vi "Set AI Channel Scale Offset (Public).vi"(7 "AI":T1=enum."DrvrVoltage_AI", 8 "error in (no error)":errorcluster, 9 "ScaleOffset":dbl, 10 "IOName":string, 11 "DAQ":refnum<class "DAQ.lvclass">) -> (0 "error out":errorcluster, 3 "DAQ":refnum<class "DAQ.lvclass">)   [LabVIEW 2017, in "DAQ.lvclass"]
doc: "Developed by Kevin Thompson\nkevin@thompsonengineering.net\n\nCopyright 2018-2020\nThompson Engineering, LLC"
uses:
  DAQ.lvclass
  DataTypes/TD AI IOName--enum.ctl
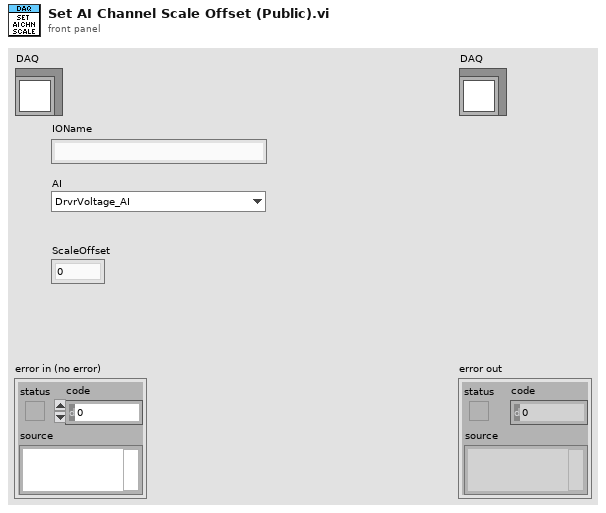
[diagram p1: front panel]
types:
  T1 = typedef "DAQ.lvclass/TD AI IOName--enum.ctl" = enum16{"DutVoltage_AI", "DrvrVoltage_AI", "DutSeriesResVoltage_AI", "DutInputCurrent_AI", "DutOutputCurrent_AI", "DutTemperature_AI"}
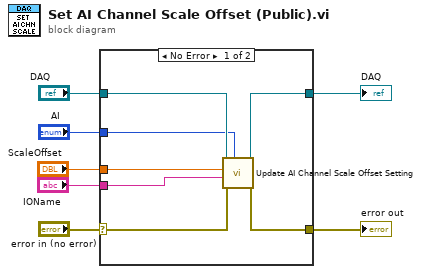
[diagram p0: block diagram]
diagram:
  n1 = case shown="No Error" "error in (no error)" {
    selector: "error in (no error)" -> [w14 w16]
    tunnel: [w13 w16] -> w6
    tunnel: [w11 w15] -> w4
    tunnel: "DAQ" -> [w12 w15]
    tunnel: "AI" -> [w10 _]
    tunnel: "ScaleOffset" -> [w9 _]
    tunnel: "IOName" -> [w8 _]
    frame No Error {
      n2 = call "Update AI Channel Scale Offset Setting.vi"("IOName (enum)"=w10, "error in (no error)"=w14, "Name"=w8, "ScaleOffset"=w9, "DAQ"=w12) -> ("error out"=w13:errorcluster, "DAQ"=w11:refnum<class "DAQ.lvclass">)  [unwired: 4 in, 1 out]
    }
    frame Error {
    }
  }
  "error out" <- w6
  "DAQ" <- w4
